vi "Motor Power.vi"() -> ()   [LabVIEW 2018]
panel:
  in  "Max_Climb_Power":dbl
  in  "Spare_Power":dbl
  in  "Vacuum_Pump_Power":dbl
  in  "Elevator_Power":dbl
  in  "Lower_Intake_Power":dbl
  in  "Upper_Intake_Power":dbl
  in  "Drive_Left_Side_Power":dbl
  in  "Drive_Right_Side_Power":dbl
  in  "Auto_Stow_Sequence":dbl
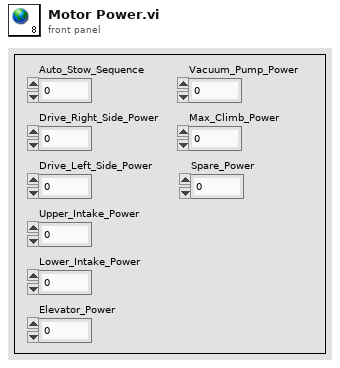
[diagram p1: front panel]
diagram:
